vi "Read_enqueueOptions.vi"(8 "error in (no error)":errorcluster, 11 "TcpServerTel in":refnum<class "TcpServerTel.lvclass">) -> (0 "error out":errorcluster, 2 "EnqueueOptions":T1, 3 "TcpServerTel out":refnum<class "TcpServerTel.lvclass">)   [LabVIEW 2018, in "TcpServerTel.lvclass"]
doc: "Read enqueue options to add new elements into telemetry queue."
uses:
  TcpServerTel.lvclass
  typedef/enqueueOptionsTypeDef.ctl
  TcpServerTel.lvclass/TcpServerTel.ctl
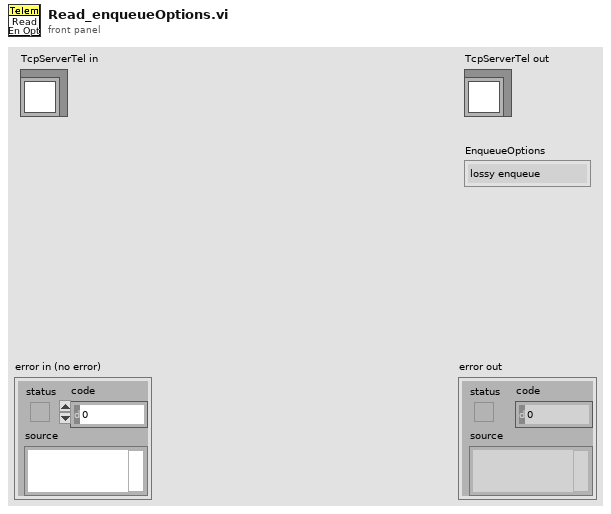
[diagram p1: front panel]
types:
  T1 = typedef "TcpServerTel.lvclass/enqueueOptionsTypeDef.ctl" = enum16{"lossy enqueue", "normal queueu"}
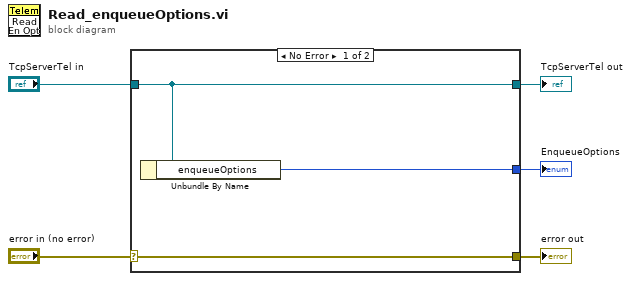
[diagram p0: block diagram]
diagram:
  n1 = case shown="No Error" "error in (no error)" {
    selector: "error in (no error)" -> [w8 w9]
    tunnel: [w8 w9] -> w4
    tunnel: [w7 w10] -> w2
    tunnel: "TcpServerTel in" -> [w7 w10]
    tunnel: [w6 _] -> w1
    frame No Error {
      n2 = Unbundle By Name(w7) -> ("enqueueOptions"=w6:T1)
    }
    frame Error {
    }
  }
  "error out" <- w4
  "TcpServerTel out" <- w2
  "EnqueueOptions" <- w1
